vi "resources list.vi"(8 "error in":errorcluster, 10 "server id":i32, 11 "message json":string) -> (0 "error out":errorcluster, 3 "response":string)   [LabVIEW 2020, in "MCP Server.lvlib"]
uses:
  MCP Server.lvlib
  add47c8a-c97f-485a-bac8-35d996f0c1d8.vi
  <vilib>/JDP Science/JSONtext/Variant to JSON Text.vi
  <vilib>/JDP Science/JSONtext/support/Format JSON Array Text.vi
  <vilib>/JDP Science/JSONtext/support/Format JSON Object.vi
  <vilib>/JDP Science/JSONtext/LVClass Serializer/JSONtext LVClass Serializer.lvclass
  <vilib>/JDP Science/JSONtext/JSONtext.lvlib
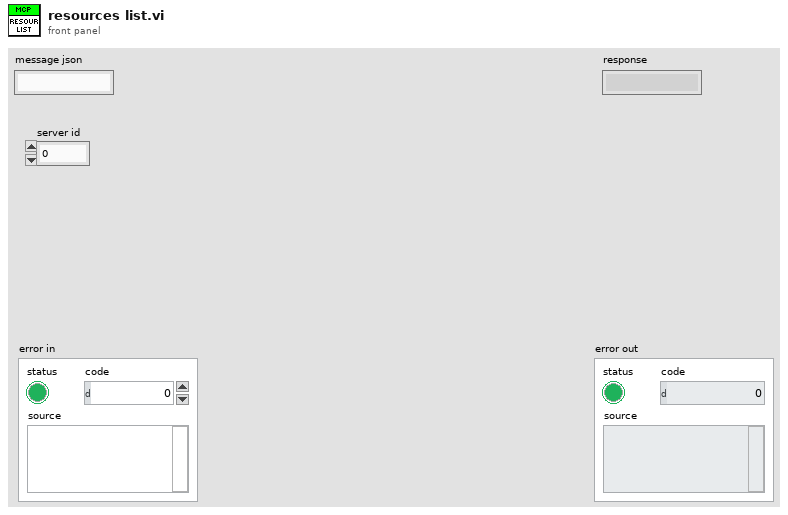
[diagram p1: front panel]
types:
  T1 = typedef "MCP Server.lvlib/resource data.ctl" = cluster{"uri":string, "name":string, "description":string, "mimeType":string, "file path":path}
  T2 = cluster{"uri":string, "name":string, "description":string, "mimeType":string}
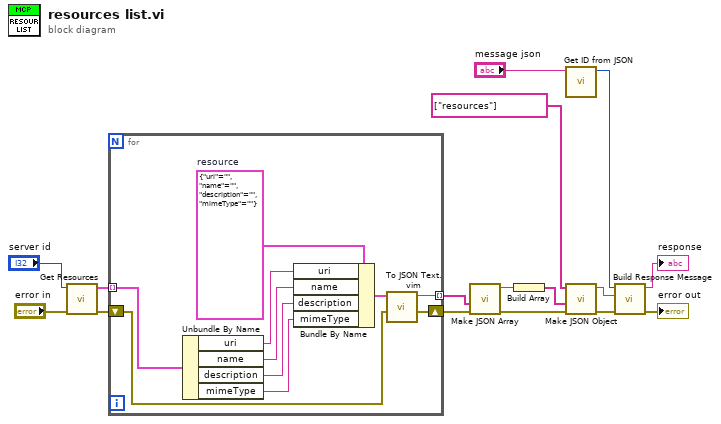
[diagram p0: block diagram]
diagram:
  n1 = call "Get Resources.vi"("error in (no error)"="error in", "id"="server id") -> ("error out"=w9:errorcluster, "resources"=w10:T1[])  [unwired: 8 in]
  n2 = for {
    tunnel: w10 -> [w25] mode=indexing
    tunnel: [w19] -> w6 mode=indexing
    shift-right: [w18] -> w8
    shift-left: w9 -> [w17]
    w26 = T2 {"uri"="", "name"="", "description"="", "mimeType"=""}  # resource
    n3 = Unbundle By Name(w25) -> ("uri"=w24:string, "name"=w23:string, "description"=w22:string, "mimeType"=w21:string)
    n4 = Bundle By Name(cluster=w26, "uri"=w24, "name"=w23, "description"=w22, "mimeType"=w21) -> (w20:T2)
    n5 = call "To JSON Text.vim"("error in (no error)"=w17, "Anything"=w20) -> ("error out"=w18:errorcluster, "<JSON>"=w19:string)  [unwired: 8 in]
  }
  n6 = call <vilib>:"Make JSON Array.vi"("error in (no error)"=w8, "JSON Elements"=w6) -> ("error out"=w7:errorcluster, "<JSON>"=w3:string)  [unwired: 8 in]
  n7 = Build Array(w3) -> (w2:string[])
  n8 = call "Get ID from JSON.vi"("message json"="message json") -> ("Data out"=w14:i32)  [unwired: 10 in]
  n9 = call <vilib>:"Make JSON Object.vi"("error in (no error)"=w7, "JSON Items"=w2, "Item Names"=string[] ["resources"]) -> ("error out"=w5:errorcluster, "<JSON>"=w1:string)  [unwired: 7 in]
  n10 = call "Build Response Message.vi"("error in (no error)"=w5, "Result content"=w1, "message id in"=w14) -> ("error out"=→"error out":errorcluster, "MCP message out"=→"response":string)  [unwired: 7 in]
